vi "setCameraName.vi"(8 "error in (no error)":errorcluster, 10 "Camera":enum16{"Simulation", "Pixis", "ProEM"}(ring), 11 "WinX32Camera in":refnum<class "WinX32Camera.lvclass">) -> (0 "error out":errorcluster, 3 "WinX32Camera out":refnum<class "WinX32Camera.lvclass">)   [LabVIEW 2011, in "WinX32Camera.lvclass"]
uses:
  WinX32Camera.lvclass
  WinX32Camera.lvclass/WinX32Camera.ctl
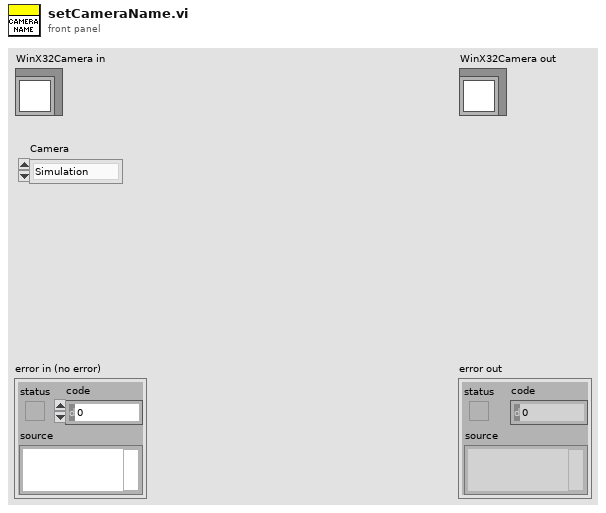
[diagram p1: front panel]
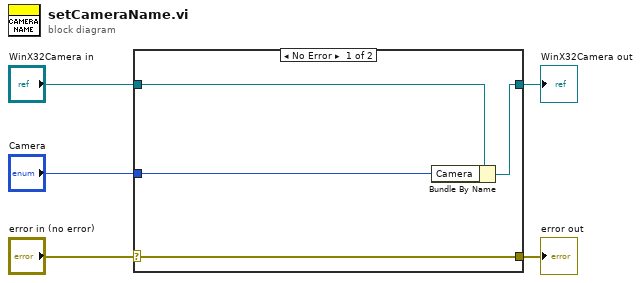
[diagram p0: block diagram]
diagram:
  n1 = case shown="No Error" "error in (no error)" {
    selector: "error in (no error)" -> [w9 w10]
    tunnel: [w9 w10] -> w4
    tunnel: [w7 w11] -> w2
    tunnel: "WinX32Camera in" -> [w8 w11]
    tunnel: "Camera" -> [w6 _]
    frame No Error {
      n2 = Bundle By Name(cluster=w8, "Camera"=w6) -> (w7:refnum<class "WinX32Camera.lvclass">)
    }
    frame Error {
    }
  }
  "error out" <- w4
  "WinX32Camera out" <- w2
